vi "perpheralsInitialise.vi"(6 "Legend":T2, 8 "PeripheralsMasterControl":T1, 9 "Cols":u8, 10 "Rows":u8, 11 "GraphPeripheralsIn":T3[][](array[typedef])) -> (3 "GraphPeripheralsOut":T3[][](array[typedef]))   [LabVIEW 2013]
uses:
  graphPeripherals.ctl
  Master_Legend.ctl
  MasterPeripherals.ctl
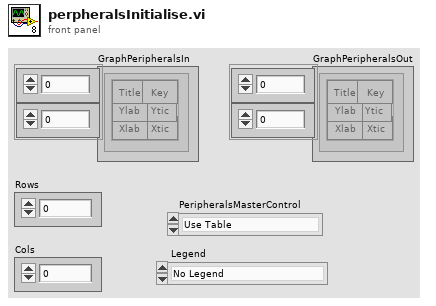
[diagram p1: front panel]
types:
  T1 = typedef "MasterPeripherals.ctl" = enum16{"Use Table", "Titles On", "Edges Only", "All Off"}
  T2 = typedef "Master_Legend.ctl" = enum16{"No Legend", "Single Legend Below table", "Legend as per array"}
  T3 = typedef "graphPeripherals.ctl" = cluster{"title":bool, "key":bool, "Xtic":bool, "Ytic":bool, "Xlab":bool, "Ylab":bool}
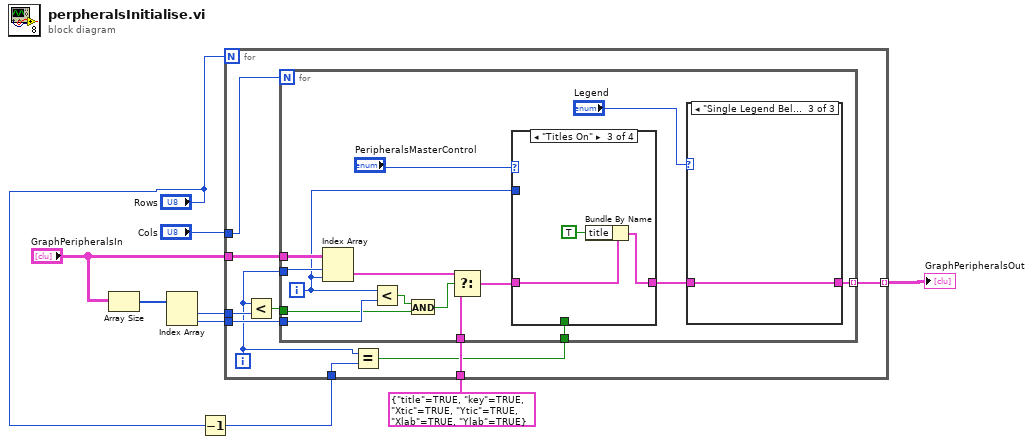
[diagram p0: block diagram]
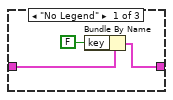
[diagram p2: hidden frame]
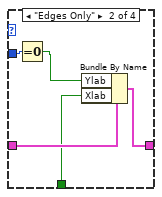
[diagram p5: hidden frame]
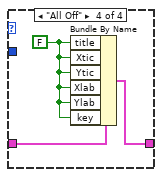
[diagram p6: hidden frame]
diagram:
  n1 = Array Size(array="GraphPeripheralsIn") -> (size(s)=w6:i32[])
  n2 = Index Array(array=w6) -> (element #1=w7:i32, element #2=w8:i32)  [unwired: 2 in]
  n3 = Decrement(x="Rows") -> (x-1=w1:u8)
  n4 = for {
    N: "Rows" -> [_]
    tunnel: "Cols" -> [w19]
    tunnel: "GraphPeripheralsIn" -> [w18]
    tunnel: [w17] -> w3 mode=indexing
    tunnel: w7 -> [w16]
    tunnel: w8 -> [w15]
    tunnel: T3 {"title"=TRUE, "key"=TRUE, "Xtic"=TRUE, "Ytic"=TRUE, "Xlab"=TRUE, "Ylab"=TRUE} ("Peripherals") -> [w13]
    tunnel: w1 -> [w12]
    i -> [w11]
    n5 = Less?(x=w11, y=w16) -> (x < y?=w14:bool)
    n6 = Equal?(x=w11, y=w12) -> (x = y?=w10:bool)
    n7 = for {
      N: w19 -> [_]
      tunnel: w18 -> [w34]
      tunnel: w11 -> [w33]
      tunnel: [w21] -> w17 mode=indexing
      tunnel: w15 -> [w32]
      tunnel: w14 -> [w30]
      tunnel: w13 -> [w27]
      tunnel: w10 -> [w24]
      i -> [w25]
      n8 = Index Array(array=w34, index (row)=w33, index (col)=w25) -> (element=w28:T3)
      n9 = Less?(x=w25, y=w32) -> (x < y?=w31:bool)
      n10 = And(x=w31, y=w30) -> (x .and. y?=w29:bool)
      n11 = Select(t=w28, s=w29, f=w27) -> (s? t:f=w26:T3)
      n12 = case shown="\"Titles On\"" "PeripheralsMasterControl" {
        tunnel: [w40 w41 w47 w50] -> w22
        tunnel: w26 -> [w40 w44 w48 w51]
        tunnel: w25 -> [_ w45 _ _]
        tunnel: w24 -> [_ w42 _ _]
        frame "Use Table", Default {
        }
        frame "Edges Only" {
          n13 = Equal To 0?(x=w45) -> (x = 0?=w43:bool)
          n14 = Bundle By Name(cluster=w44, "Ylab"=w43, "Xlab"=w42) -> (w41:T3)
        }
        frame "Titles On" {
          n15 = Bundle By Name(cluster=w48, "title"=TRUE) -> (w47:T3)
        }
        frame "All Off" {
          w49 = FALSE ("title")
          n16 = Bundle By Name(cluster=w51, "title"=w49, "Xtic"=w49, "Ytic"=w49, "Xlab"=w49, "Ylab"=w49, "key"=w49) -> (w50:T3)
        }
      }
      n17 = case shown="\"Single Legend Below table\"" "Legend" {
        tunnel: w22 -> [w37 w38 w39]
        tunnel: [w36 w38 w39] -> w21
        frame "No Legend" {
          n18 = Bundle By Name(cluster=w37, "key"=FALSE) -> (w36:T3)
        }
        frame "Legend as per array" {
        }
        frame "Single Legend Below table" {
        }
      }
    }
  }
  "GraphPeripheralsOut" <- w3
